vi "Get Server State UE.vi"(11 "Template Server in":refnum<class "MeasurementService_Template.lvclass">) -> (2 "Server Internal State UE":refnum<user-event>, 3 "Template Server out":refnum<class "MeasurementService_Template.lvclass">)   [LabVIEW 2020, in "LoadRegulation.lvlib" / "MeasurementService_Template.lvclass"]
uses:
  MeasurementService_Template.lvclass
  typeDefs/Server State Data.ctl
  MeasurementService_Template.lvclass/MeasurementService_Template.ctl
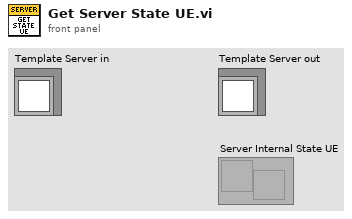
[diagram p1: front panel]
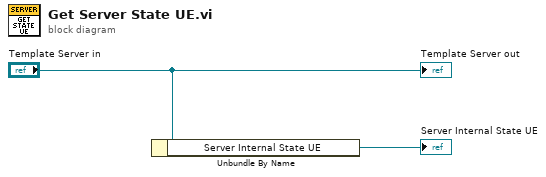
[diagram p0: block diagram]
diagram:
  n1 = Unbundle By Name("Template Server in") -> ("Server Internal State UE"=→"Server Internal State UE":refnum<user-event>)
  "Template Server out" <- "Template Server in"
